vi "MAIN_STANDALONE.vi"() -> ()   [LabVIEW 2019]
uses:
  LVPROJ_CREAR BANDEJAS/Type_defs/Data_Bandeja.ctl
  LVPROJ_CONFIG_ESTACION/Type_defs/Coordenadas_estacion.ctl
  SHARED VI'S/SHARED VI'S.lvlib
  LVPROJ_MOVIMIENTO_CABEZAL/LABVIEW_MOVIMIENTO/MOVIMIENTO CABEZAL/Typedefs/Comandos.ctl
  LVPROJ_MOVIMIENTO_CABEZAL/LABVIEW_MOVIMIENTO/MOVIMIENTO CABEZAL/Typedefs/Estados_arduino.ctl
  <vilib>/Instr/_visa.llb/VISA Configure Serial Port (Instr).vi
  TYPE'S DEF/State_QR.ctl
  TYPE'S DEF/OUTPUTS_lecturaQR.ctl
  TYPE'S DEF/INPUT LECTURA_QR.ctl
panel:
  out "QR pendientes":u32
  out "FINAL QR?":bool
  in  "Tab Control":T1(tab)
  in  "ENVIAR PARAMETROS DE LECTURA":bool
  in  "DETENER TEST":bool
  in  "EXIT":bool
  in  "COMENZAR LECTURA":bool
  in  "LECTURA QR INPUT":T2={"COORD X"=0, "COORD  Y"=0, "NºASICS"=1, "SELECCIÓN DE BANDEJA"=enum."BANDEJA ENTRADA", "CONTEO QR"=0}
  out "INDICADORES DE TEST":T3
  out "Configuracion Estación":T4={"Coordenadas_estacion"={"Coord.Bandeja entrada"={"Coord. X0 entrada"=0, "Coord. Y0 entrada "=0, "Altura Z entrada"=0}, "Coord.Bandeja OK"={"Coord. X0 OK"=0, "Coord. Y0 OK"=0, "Altura Z OK"=0}, "Coord.Bandeja entrada FAIL"={"Coord. X0 FAIL"=0, "Coord. Y0 FAIL"=0, "Altura Z FAIL"=0}, "Coord. Socket"={"Coord. X socket"=0, "Coord. Y socket"=0, "Altura Z socket"=0}}, "Nombre Bandeja"="", "Datos bandeja"={"Nº de columnas "=0, "Nº de filas "=0, "largo"=0, "ancho"=0, "nombre"="nombre", "Paso X (en mm)"=0.0, "Paso Y (en mm)"=0.0, "DISTANCIA SUELO A CHIP  "=0.0, "Nº de celdas totales"=0, "Distancia chips bandejas contiguas"=0.0}}
  out "Error Out":errorcluster
  in  "Error In":errorcluster
  # "CELDA DE COMIENZO"
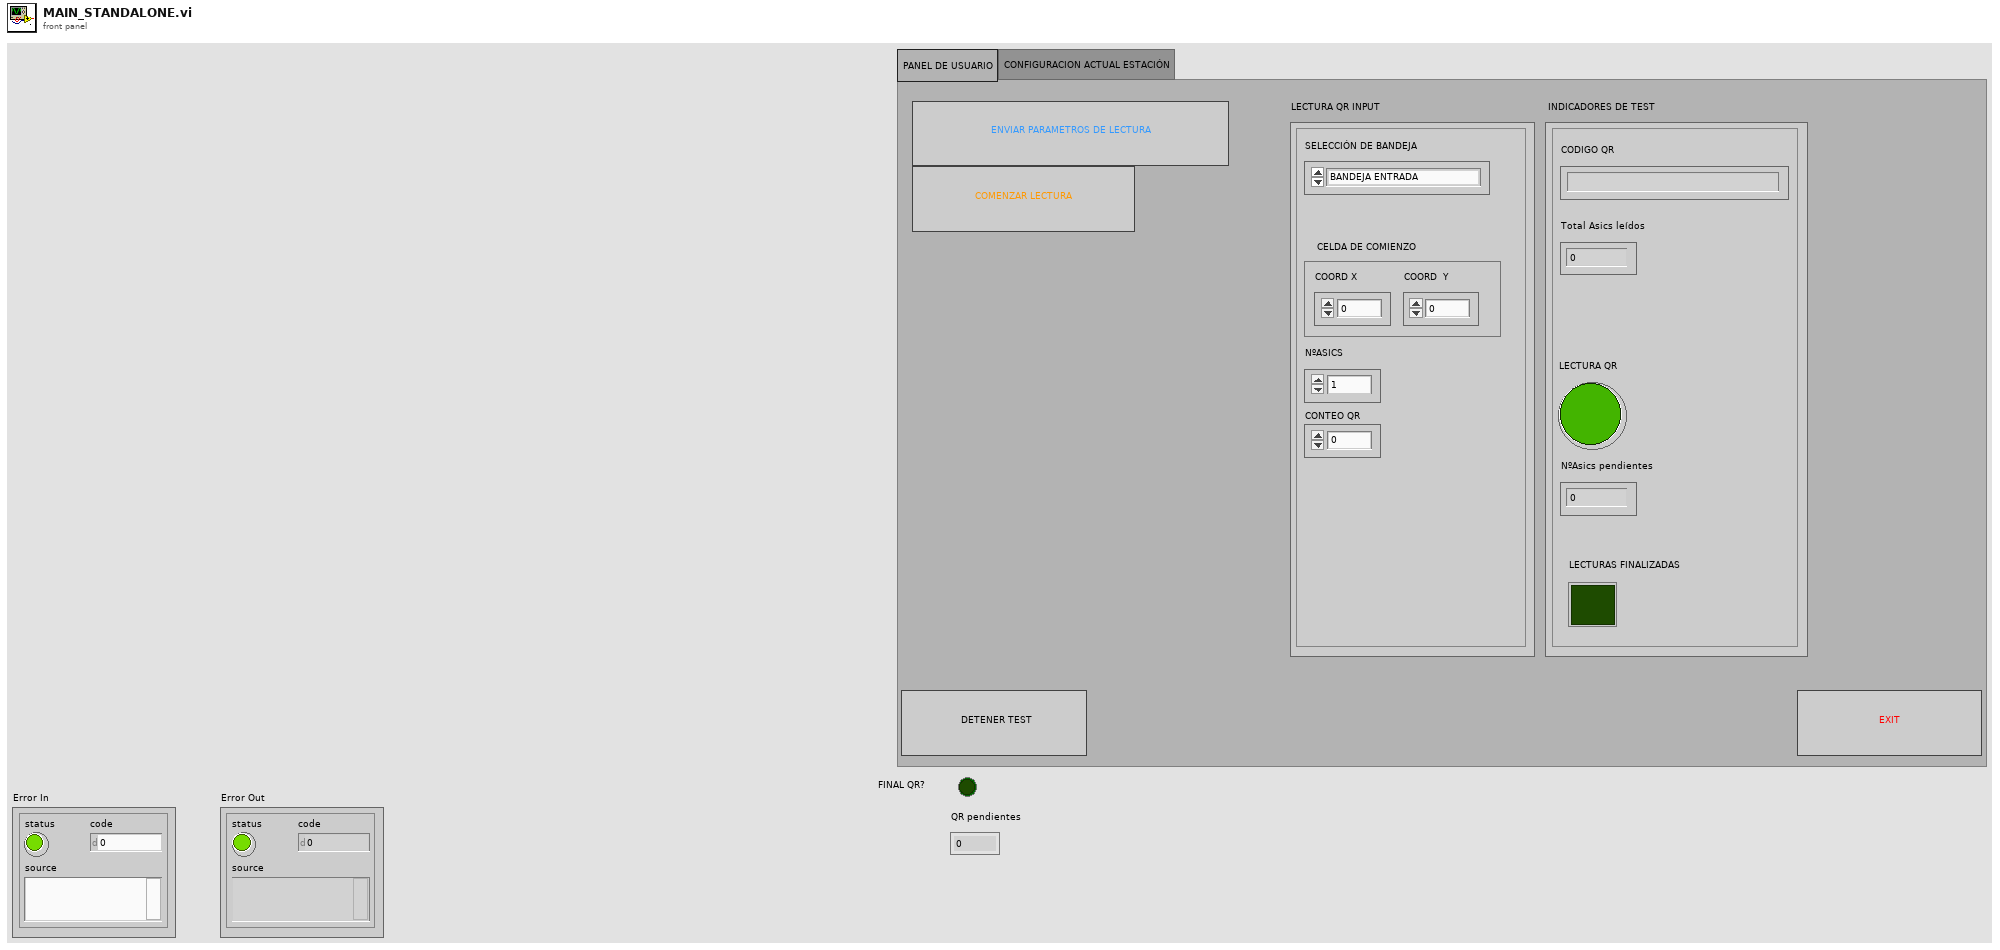
[diagram p1: front panel]
types:
  T1 = enum32{"PANEL DE USUARIO", "CONFIGURACION ACTUAL ESTACIÓN"}
  T2 = typedef "INPUT LECTURA_QR.ctl" = cluster{"COORD X":u16, "COORD  Y":u16, "NºASICS":u32, "SELECCIÓN DE BANDEJA":enum16{"BANDEJA ENTRADA", "BANDEJA OK", "BANDEJA NOK"}, "CONTEO QR":u32}
  T3 = typedef "OUTPUTS_lecturaQR.ctl" = cluster{"CODIGO QR":string, "LECTURA QR":bool, "LECTURAS FINALIZADAS":bool, "Total Asics leídos":u32, "NºAsics pendientes":u32}
  T4 = typedef "Configuracion_estación.ctl" = cluster{"Coordenadas_estacion":T5, "Nombre Bandeja":string, "Datos bandeja":T6}
  T5 = typedef "Coordenadas_estacion.ctl" = cluster{"Coord.Bandeja entrada":cluster{"Coord. X0 entrada":u32, "Coord. Y0 entrada ":u32, "Altura Z entrada":u32}, "Coord.Bandeja OK":cluster{"Coord. X0 OK":u32, "Coord. Y0 OK":u32, "Altura Z OK":u32}, "Coord.Bandeja entrada FAIL":cluster{"Coord. X0 FAIL":u32, "Coord. Y0 FAIL":u32, "Altura Z FAIL":u32}, "Coord. Socket":cluster{"Coord. X socket":u32, "Coord. Y socket":u32, "Altura Z socket":u32}}
  T6 = typedef "Data_Bandeja.ctl" = cluster{"Nº de columnas ":u32, "Nº de filas ":u32, "largo":u32, "ancho":u32, "nombre":string, "Paso X (en mm)":dbl, "Paso Y (en mm)":dbl, "DISTANCIA SUELO A CHIP  ":dbl, "Nº de celdas totales":u16, "Distancia chips bandejas contiguas":dbl}
  T7 = typedef "State_QR.ctl" = enum16{"Init", "Wait for Event", "Init refs", "Init com", "Config estacion", "Home", "Ping_Arduino", "Coge Asic", "Enviar_config_test", "Dejar Asic", "Leer QR", "Actualizar valores", "Enviar OK Arduino", "Final de lecturas?", "Terminar", "Exit", "Error?"}
  T8 = typedef "Comandos.ctl" = enum16{"H", "FH", "FM", "FI", "FX", "FY", "FZ", "I", "OK"}
  T9 = typedef "Estados_arduino.ctl" = enum16{"2", "3", "4", "5", "6", "7", "9", "8"}
  T10 = enum16{"BANDEJA ENTRADA", "BANDEJA OK", "BANDEJA NOK"}
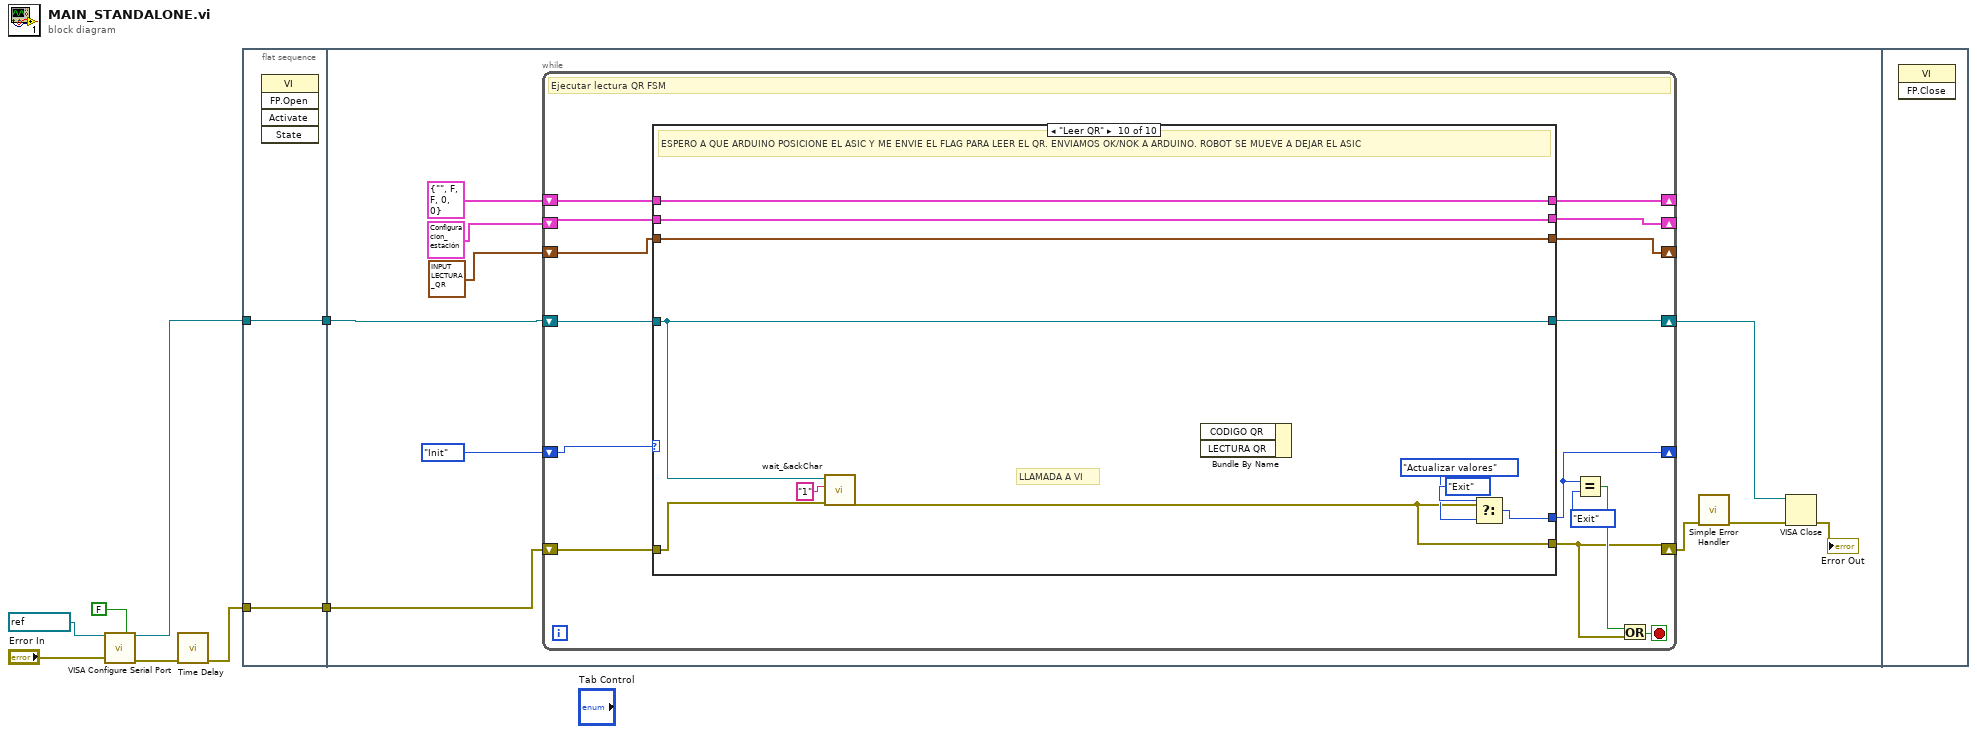
[diagram p0: block diagram]
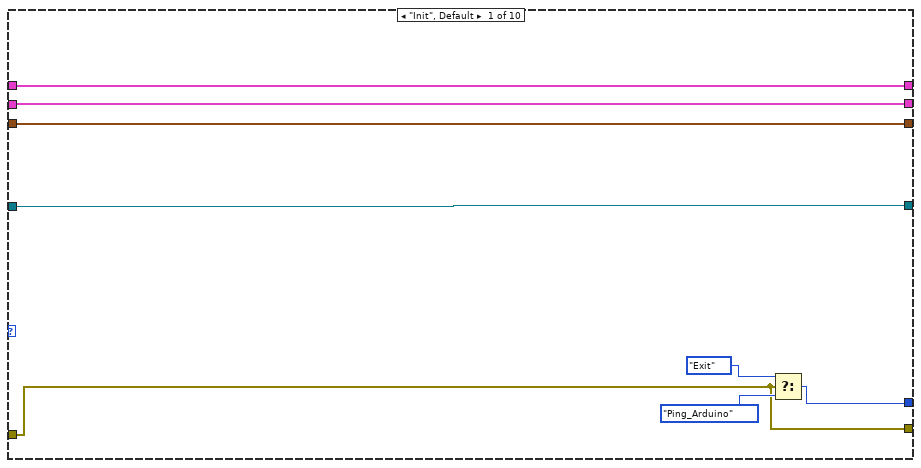
[diagram p2: hidden frame]
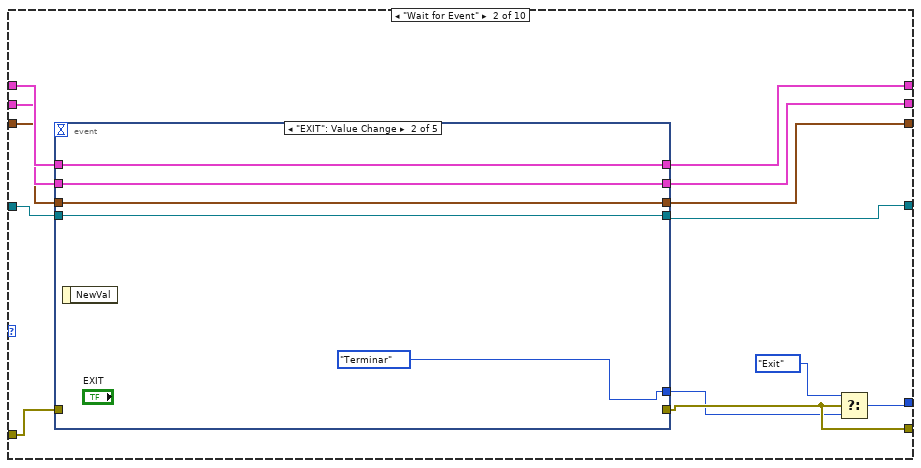
[diagram p3: hidden frame]
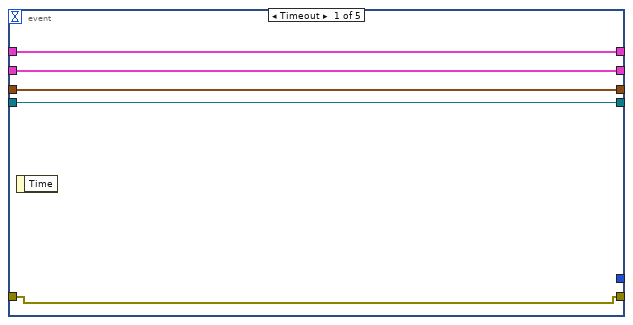
[diagram p4: hidden frame]
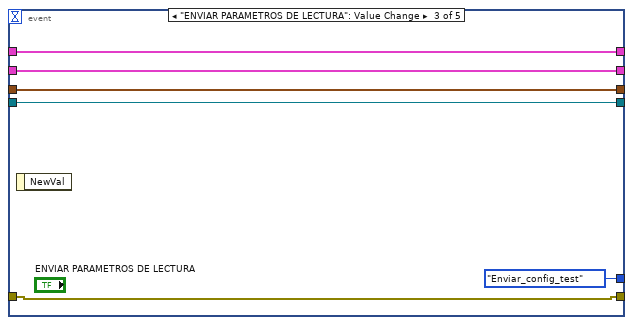
[diagram p5: hidden frame]
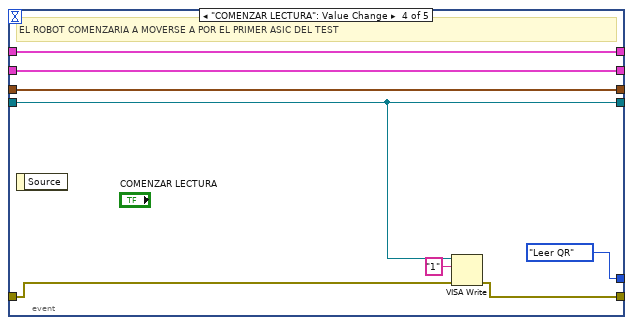
[diagram p6: hidden frame]
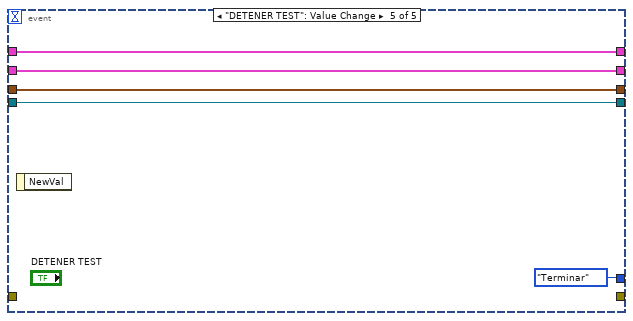
[diagram p7: hidden frame]
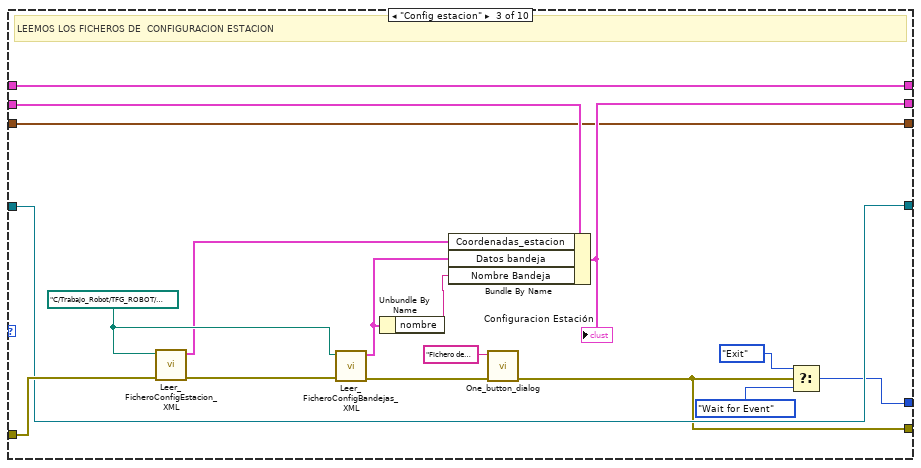
[diagram p8: hidden frame]
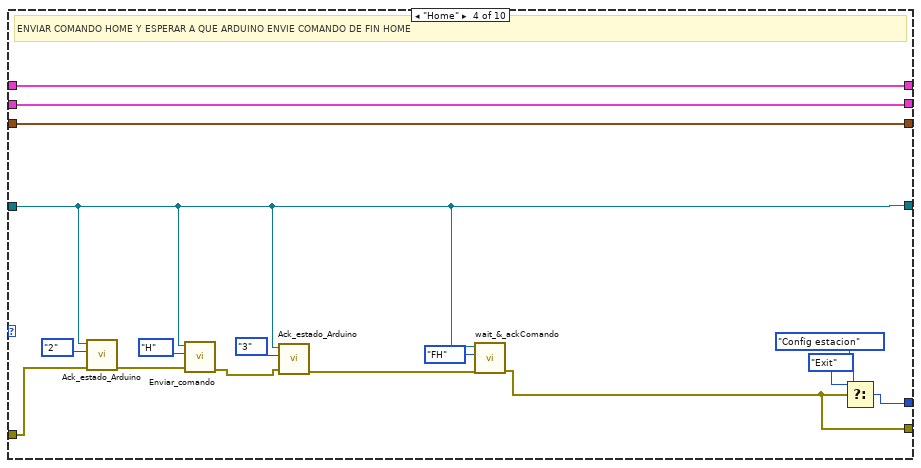
[diagram p9: hidden frame]
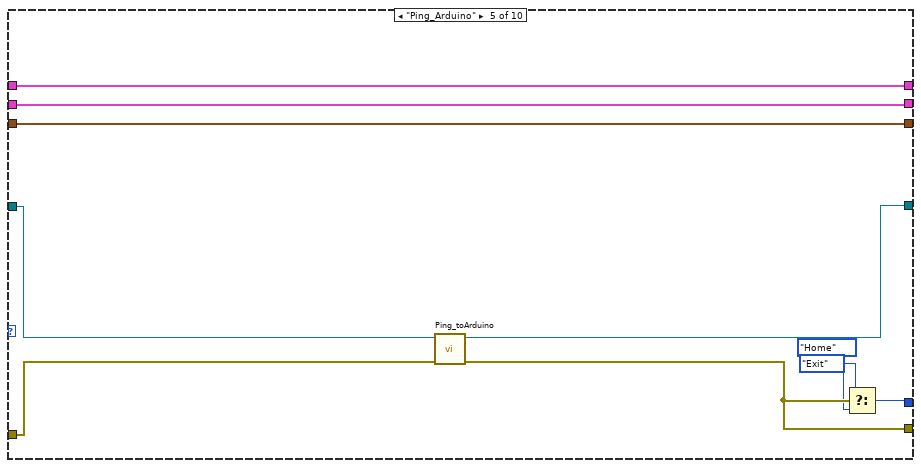
[diagram p10: hidden frame]
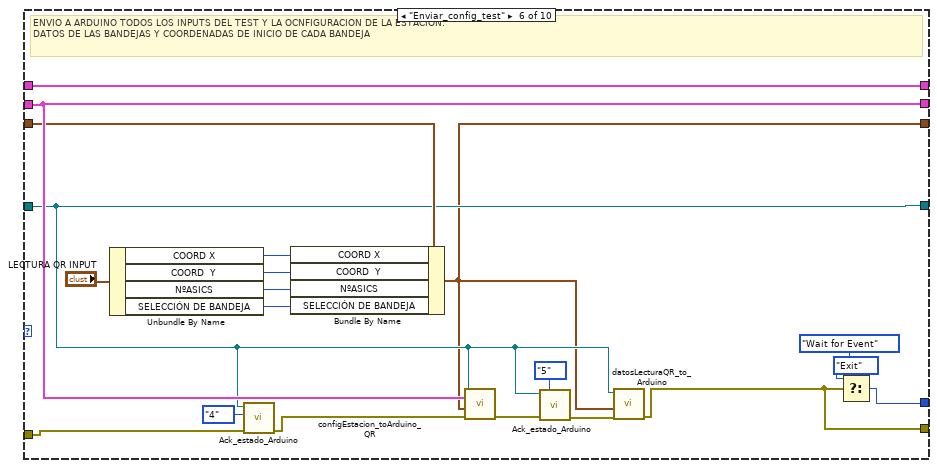
[diagram p11: hidden frame]
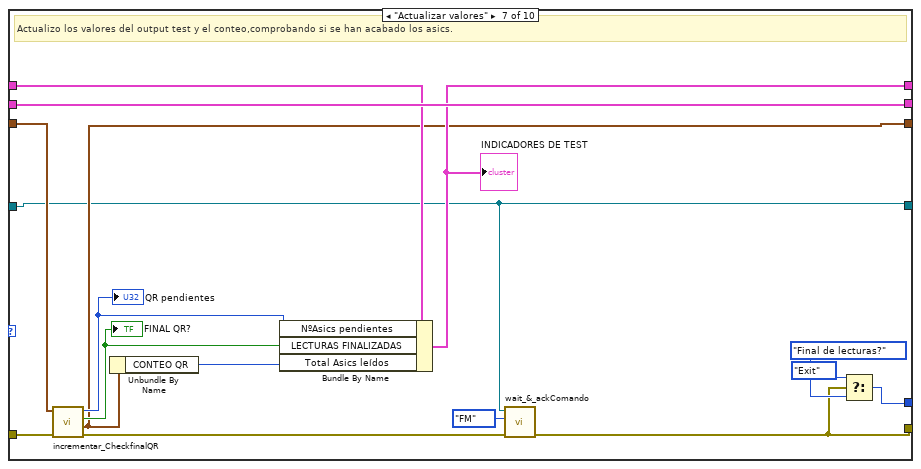
[diagram p12: hidden frame]
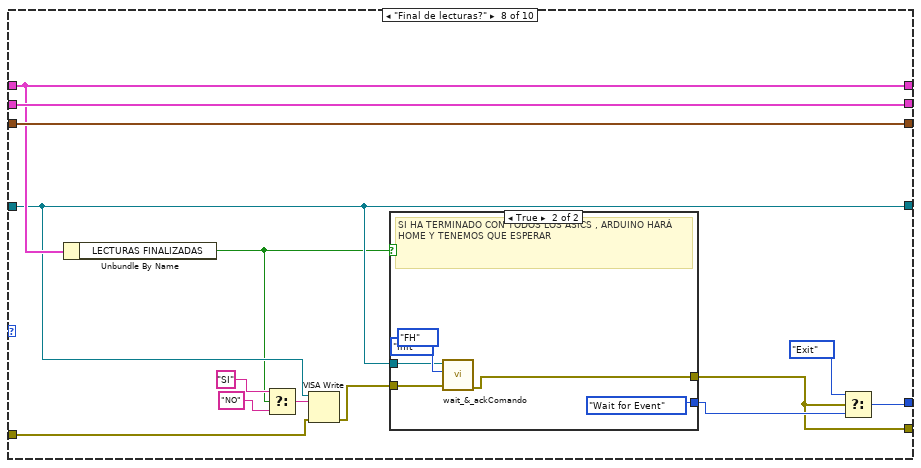
[diagram p13: hidden frame]
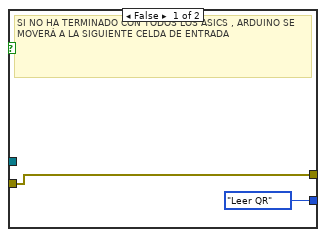
[diagram p14: hidden frame]
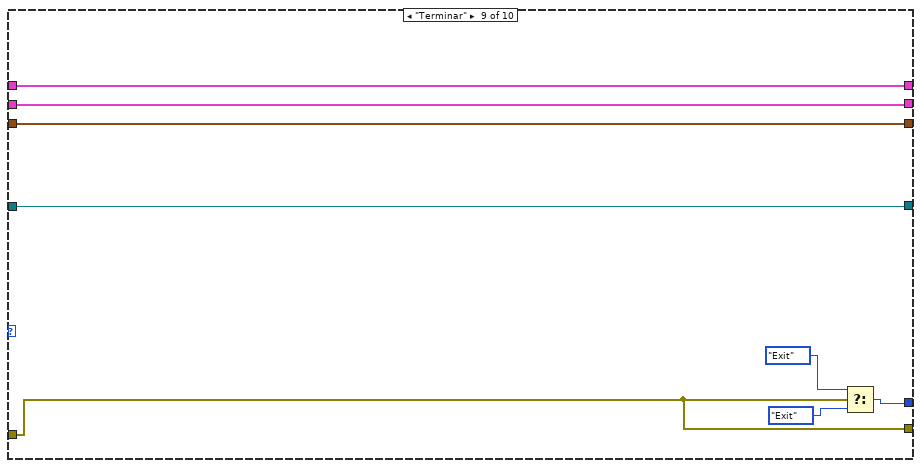
[diagram p15: hidden frame]
diagram:
  n1 = call-poly "VISA Configure Serial Port"("VISA resource name"=refnum<visa-resource-name> "COM4", "Enable Termination\nChar (T)"=FALSE ("Enable Termination\nChar (T)"), "error in (no error)"="Error In") -> ("VISA resource name out"=w1:refnum<visa-resource-name>, "error out"=w3:errorcluster)  [unwired: 11 in]
  n2 = call "Time Delay"("error in (no error)"=w3) -> ("error out"=w2:errorcluster)  [unwired: 10 in]
  n3 = flat-sequence {
    tunnel: w2 -> [w10]
    tunnel: [w10] -> w8
    tunnel: w1 -> [w9]
    tunnel: [w9] -> w7
    tunnel: w8 -> [w18]
    tunnel: w7 -> [w17]
    frame #0 {
      n4 = invoke class="VI" method="FP.Open"() -> ()  [unwired: 5 in, 5 out]
    }
    frame #1 {
      n5 = while {
        shift-right: [w30] -> w12
        shift-left: w18 -> [w34]
        shift-right: [w23] -> _
        shift-left: T2 {"COORD X"=0, "COORD  Y"=0, "NºASICS"=0, "SELECCIÓN DE BANDEJA"=enum."BANDEJA ENTRADA", "CONTEO QR"=0} ("TEST ASICS INPUT") -> [w33]
        shift-right: [w25] -> _
        shift-left: T4 {"Coordenadas_estacion"={"Coord.Bandeja entrada"={"Coord. X0 entrada"=0, "Coord. Y0 entrada "=0, "Altura Z entrada"=0}, "Coord.Bandeja OK"={"Coord. X0 OK"=0, "Coord. Y0 OK"=0, "Altura Z OK"=0}, "Coord.Bandeja entrada FAIL"={"Coord. X0 FAIL"=0, "Coord. Y0 FAIL"=0, "Altura Z FAIL"=0}, "Coord. Socket"={"Coord. X socket"=0, "Coord. Y socket"=0, "Altura Z socket"=0}}, "Nombre Bandeja"="", "Datos bandeja"={"Nº de columnas "=0, "Nº de filas "=0, "largo"=0, "ancho"=0, "nombre"="nombre", "Paso X (en mm)"=0.0, "Paso Y (en mm)"=0.0, "DISTANCIA SUELO A CHIP  "=0.0, "Nº de celdas totales"=0, "Distancia chips bandejas contiguas"=0.0}} ("Configuracion Estación") -> [w29]
        shift-right: [w27] -> w13
        shift-left: w17 -> [w28]
        shift-right: [w24] -> _
        shift-left: T3 {"CODIGO QR"="", "LECTURA QR"=FALSE, "LECTURAS FINALIZADAS"=FALSE, "Total Asics leídos"=0, "NºAsics pendientes"=0} -> [w26]
        shift-right: [w21] -> _
        shift-left: State_QR."Init" ("States_main") -> [w22]
        stop <- w32 stop-if-true
        # "Ejecutar lectura QR FSM"
        n6 = case shown="\"Leer QR\"" w22 {
          tunnel: w34 -> [w37 w50 w102 w110 w125 w136 w159 w171 w189 w203]
          tunnel: w33 -> [w39 w52 w91 w116 w126 w143 w160 w177 w191 w198]
          tunnel: [w37 w49 w87 w103 w123 w144 w151 w168 w189 w194] -> w30
          tunnel: w29 -> [w40 w54 w94 w117 w127 w145 w162 w178 w192 w199]
          tunnel: w28 -> [w38 w45 w95 w105 w124 w131 w150 w166 w190 w196]
          tunnel: [w38 w44 w95 w105 w122 w131 w150 w166 w190 w196] -> w27
          tunnel: w26 -> [w41 w56 w92 w118 w128 w146 w154 w176 w193 w200]
          tunnel: [w40 w53 w93 w117 w127 w145 w162 w178 w192 w199] -> w25
          tunnel: [w41 w55 w92 w118 w128 w146 w153 w176 w193 w200] -> w24
          tunnel: [w39 w51 w91 w116 w126 w129 w152 w177 w191 w198] -> w23
          tunnel: [w36 w46 w88 w107 w119 w137 w161 w167 w186 w197] -> w21
          frame "Init", Default {
            n7 = Select(t=State_QR."Exit" ("States_main"), s=w37, f=State_QR."Ping_Arduino" ("States_main")) -> (s? t:f=w36:T7)
          }
          frame "Wait for Event" {
            n8 = event shown="[1] \"EXIT\": Value Change" {
              selector: _ -> [_ _ _ _ _]
              dyn-events: _ -> [_ _ _ _ _]
              timeout: _ -> [_ _ _ _ _]
              tunnel: w56 -> [w61 w66 w72 w80 w85]
              tunnel: [w61 w66 w72 w80 w85] -> w55
              tunnel: w54 -> [w60 w65 w71 w79 w84]
              tunnel: [w60 w65 w71 w79 w84] -> w53
              tunnel: w52 -> [w59 w64 w70 w78 w83]
              tunnel: [w59 w64 w70 w78 w83] -> w51
              tunnel: w50 -> [w58 _ w69 w75 _]
              tunnel: [w58 _ w69 w74 _] -> w49
              tunnel: [_ State_QR."Terminar" ("States_main") State_QR."Enviar_config_test" ("States_main") State_QR."Leer QR" ("States_main") State_QR."Terminar" ("States_main")] -> w47
              tunnel: w45 -> [w57 w62 w67 w76 w81]
              tunnel: [w57 w62 w67 w76 w81] -> w44
              event Timeout {
                n9 = event-data() -> ()  [unwired: 1 in, 1 out]
              }
              event "EXIT": Value Change {
                n10 = event-data() -> ()  [unwired: 1 in, 1 out]
              }
              event "ENVIAR PARAMETROS DE LECTURA": Value Change {
                n11 = event-data() -> ()  [unwired: 1 in, 1 out]
              }
              event "COMENZAR LECTURA": Value Change {
                # "EL ROBOT COMENZARIA A MOVERSE A POR EL PRIMER ASIC DEL TEST"
                n12 = event-data() -> ()  [unwired: 1 in, 1 out]
                n13 = VISA Write(VISA resource name=w76, write buffer="1", error in (no error)=w75) -> (error out=w74:errorcluster)  [unwired: 2 out]
              }
              event "DETENER TEST": Value Change {
                n14 = event-data() -> ()  [unwired: 1 in, 1 out]
              }
            }
            n15 = Select(t=State_QR."Exit" ("States_main"), s=w49, f=w47) -> (s? t:f=w46:T7)
          }
          frame "Config estacion" {
            w100 = path "C:/Trabajo_Robot/TFG_ROBOT/CONTROL_ROBOT/LABVIEW_ROBOT_MASTER" ("XML File Path")
            # "LEEMOS LOS FICHEROS DE  CONFIGURACION ESTACION"
            n16 = call "Leer_FicheroConfigEstacion_XML.vi"("error in (no error)"=w102, "XML File Path"=w100) -> ("error out"=w101:errorcluster, "Coordenadas_estacion"=w99:T5)  [unwired: 8 in]
            n17 = call "Leer_FicheroConfigBandejas_XML.vi"("error in (no error)"=w101, "XML File Path"=w100) -> ("error out"=w96:errorcluster, "Datos bandeja"=w98:T6)  [unwired: 8 in]
            n18 = Unbundle By Name(w98) -> ("nombre"=w97:string)
            n19 = Bundle By Name(cluster=w94, "Coordenadas_estacion"=w99, "Datos bandeja"=w98, "Nombre Bandeja"=w97) -> (w93:T4)
            "Configuracion Estación" <- w93
            n20 = call "One_button_dialog.vi"("error in (no error)"=w96, "message"="Fichero de configuración cargado correctamente.") -> ("error out"=w87:errorcluster)  [unwired: 9 in]
            n21 = Select(t=State_QR."Exit" ("States_main"), s=w87, f=State_QR."Wait for Event" ("States_main")) -> (s? t:f=w88:T7)
          }
          frame "Home" {
            # "ENVIAR COMANDO HOME Y ESPERAR A QUE ARDUINO ENVIE COMANDO DE FIN HOME"
            n22 = call "Ack_estado_Arduino.vi"("error in (no error)"=w110, "Enum"=Estados_arduino."2", "VISA resource name"=w105) -> ("error out"=w115:errorcluster)  [unwired: 6 in, 2 out]
            n23 = call "Enviar_comando.vi"("error in (no error)"=w115, "Enum"=Comandos."H", "VISA resource name"=w105) -> ("error out"=w111:errorcluster)  [unwired: 6 in, 2 out]
            n24 = call "Ack_estado_Arduino.vi"("error in (no error)"=w111, "Enum"=Estados_arduino."3", "VISA resource name"=w105) -> ("error out"=w106:errorcluster)  [unwired: 6 in, 2 out]
            n25 = call "wait_&_ackComando.vi"("error in (no error)"=w106, 10:Comandos."FH", "VISA Refnum in"=w105) -> ("error out"=w103:errorcluster)  [unwired: 7 in, 1 out]
            n26 = Select(t=State_QR."Exit" ("States_main"), s=w103, f=State_QR."Config estacion" ("States_main")) -> (s? t:f=w107:T7)
          }
          frame "Ping_Arduino" {
            n27 = call "Ping_toArduino.vi"("error in (no error)"=w125, "VISA Refnum in"=w124) -> ("error out"=w123:errorcluster, "VISA Refnum out"=w122:refnum<visa-resource-name>)  [unwired: 7 in, 1 out]
            n28 = Select(t=State_QR."Exit" ("States_main"), s=w123, f=State_QR."Home" ("States_main")) -> (s? t:f=w119:T7)
          }
          frame "Enviar_config_test" {
            # "ENVIO A ARDUINO TODOS LOS INPUTS DEL TEST Y LA OCNFIGURACION DE LA ESTACIÓN:\nDATOS DE LAS BANDEJAS Y COORDENADAS DE INICIO DE CADA BANDEJA"
            n29 = Unbundle By Name("LECTURA QR INPUT") -> ("COORD X"=w142:u16, "COORD  Y"=w141:u16, "NºASICS"=w140:u32, "SELECCIÓN DE BANDEJA"=w139:T10)
            n30 = call "Ack_estado_Arduino.vi"("error in (no error)"=w136, "Enum"=Estados_arduino."4", "VISA resource name"=w131) -> ("error out"=w134:errorcluster)  [unwired: 6 in, 2 out]
            n31 = Bundle By Name(cluster=w143, "COORD X"=w142, "COORD  Y"=w141, "NºASICS"=w140, "SELECCIÓN DE BANDEJA"=w139) -> (w129:T2)
            n32 = call "configEstacion_toArduino_QR.vi"("error in (no error)"=w134, "LECTURA QR INPUT"=w129, "Configuracion Estación"=w145, "VISA resource name"=w131) -> ("error IO"=w133:errorcluster)  [unwired: 5 in, 2 out]
            n33 = call "Ack_estado_Arduino.vi"("error in (no error)"=w133, "Enum"=Estados_arduino."5", "VISA resource name"=w131) -> ("error out"=w132:errorcluster)  [unwired: 6 in, 2 out]
            n34 = call "datosLecturaQR_to_Arduino.vi"("error in (no error)"=w132, "LECTURA QR INPUT"=w129, "VISA resource name"=w131) -> ("error IO"=w144:errorcluster)  [unwired: 7 in, 1 out]
            n35 = Select(t=State_QR."Exit" ("States_main"), s=w144, f=State_QR."Wait for Event" ("States_main")) -> (s? t:f=w137:T7)
          }
          frame "Actualizar valores" {
            # "Actualizo los valores del output test y el conteo,comprobando si se han acabado los asics."
            n36 = call "incrementar_CheckfinalQR.vi"("error in (no error)"=w159, "TEST ASICS INPUT"=w160) -> ("error out"=w158:errorcluster, "output cluster"=w152:T2, "FINAL ASICS??"=w156:bool, "Asics pendientes"=w157:u32)  [unwired: 6 in]
            "FINAL QR?" <- w156
            "QR pendientes" <- w157
            n37 = Unbundle By Name(w152) -> ("CONTEO QR"=w155:u32)
            n38 = Bundle By Name(cluster=w154, "NºAsics pendientes"=w157, "LECTURAS FINALIZADAS"=w156, "Total Asics leídos"=w155) -> (w153:T3)
            "INDICADORES DE TEST" <- w153
            n39 = call "wait_&_ackComando.vi"("error in (no error)"=w158, 10:Comandos."FM", "VISA Refnum in"=w150) -> ("error out"=w151:errorcluster)  [unwired: 7 in, 1 out]
            n40 = Select(t=State_QR."Exit" ("States_main"), s=w151, f=State_QR."Final de lecturas?" ("States_main")) -> (s? t:f=w161:T7)
          }
          frame "Final de lecturas?" {
            (unwired) State_QR."Init" ("States_main")
            n41 = Unbundle By Name(w176) -> ("LECTURAS FINALIZADAS"=w165:bool)
            n42 = Select(t="SI", s=w165, f="NO") -> (s? t:f=w173:string)
            n43 = VISA Write(VISA resource name=w166, write buffer=w173, error in (no error)=w171) -> (error out=w172:errorcluster)  [unwired: 2 out]
            n44 = case shown="True" w165 {
              tunnel: w172 -> [w180 w185]
              tunnel: [w180 w183] -> w168
              tunnel: [State_QR."Leer QR" ("States_main") State_QR."Wait for Event" ("States_main")] -> w170
              tunnel: w166 -> [_ w181]
              frame False {
                # "SI NO HA TERMINADO CON TODOS LOS ASICS , ARDUINO SE MOVERÁ A LA SIGUIENTE CELDA DE ENTRADA"
              }
              frame True {
                # "SI HA TERMINADO CON TODOS LOS ASICS , ARDUINO HARÁ HOME Y TENEMOS QUE ESPERAR"
                n45 = call "wait_&_ackComando.vi"("error in (no error)"=w185, 10:Comandos."FH", "VISA Refnum in"=w181) -> ("error out"=w183:errorcluster)  [unwired: 7 in, 1 out]
              }
            }
            n46 = Select(t=State_QR."Exit", s=w168, f=w170) -> (s? t:f=w167:T7)
          }
          frame "Terminar" {
            n47 = Select(t=State_QR."Exit" ("y"), s=w189, f=State_QR."Exit" ("y")) -> (s? t:f=w186:T7)
          }
          frame "Leer QR" {
            # "LLAMADA A VI"
            # "ESPERO A QUE ARDUINO POSICIONE EL ASIC Y ME ENVIE EL FLAG PARA LEER EL QR. ENVIAMOS OK/NOK A ARDUINO. ROBOT SE MUEVE A DEJAR EL ASIC"
            n48 = call "wait_&ackChar.vi"("error in (no error)"=w203, "caracter"="1", "VISA Refnum in"=w196) -> ("error out"=w194:errorcluster)  [unwired: 7 in, 1 out]
            n49 = Bundle By Name() -> ()  [unwired: 3 in, 1 out]
            n50 = Select(t=State_QR."Exit" ("States_main"), s=w194, f=State_QR."Actualizar valores" ("States_main")) -> (s? t:f=w197:T7)
          }
        }
        n51 = Equal?(x=w21, y=State_QR."Exit") -> (x = y?=w35:bool)
        n52 = Or(x=w35, y=w30) -> (x .or. y?=w32:bool)
      }
      n53 = call <vilib>:"Simple Error Handler.vi"("error in (no error)"=w12) -> ("error out"=w11:errorcluster)  [unwired: 4 in, 4 out]
      n54 = VISA Close(VISA resource name=w13, error in (no error)=w11) -> (error out=→"Error Out":errorcluster)
    }
    frame #2 {
      n55 = invoke class="VI" method="FP.Close"() -> ()  [unwired: 3 in, 3 out]
    }
  }
